vi "PCI1220电动缸速度设置.vi"(10 "Change Velocity":dbl=10000.0, 11 "AxisHandle IN":u32) -> (3 "AxisHandle OUT":u32)   [LabVIEW 2013]
panel:
  out "error out":errorcluster
  out "ReturnValue":u32
  out "输出变量":dbl
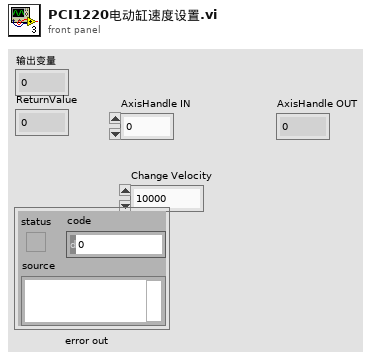
[diagram p1: front panel]
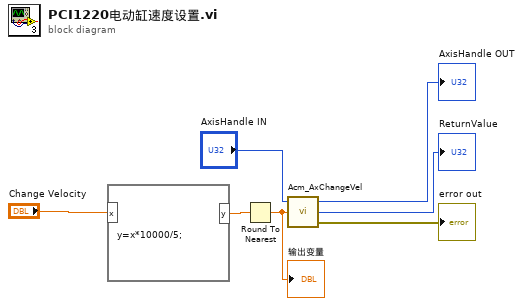
[diagram p0: block diagram]
diagram:
  n1 = formula code="y=x*10000/5;"("x"="Change Velocity") -> ("y"=w3:dbl)
  n2 = Round To Nearest(number=w3) -> (nearest integer value=w2:dbl)
  "输出变量" <- w2
  n3 = call <userlib>:"Acm_AxChangeVel.vi"("NewVelocity"=w2, "AxisHandle"="AxisHandle IN") -> ("Error Output"=→"error out":errorcluster, "ReturnValue"=→"ReturnValue":u32, "AxisHandle 2"=→"AxisHandle OUT":u32)  [unwired: 1 in]
